vi "Allowed Frequency Mask.vi"() -> ()   [LabVIEW 2010]
panel:
  out "Array":u8[](array[numeric])=[0, 0, 1, 255, 0, 0, 0, 0] format="%.0x"
  out "Allowed Frequencies":u32[](array[numeric])=[70, 75, 80, 85, 90, 95, 100, 110, 120]
  out "Byte #":u8=3
  out "Selected Frequency":u32=70
  in  "ProgramFrequencyIndex":u8=23
  in  "Allowed Frequencies Table {Hz}":cluster{"Bin":u32[], "index":u32[]}[](array[cluster])=[{"Bin"=[14, 12, 10, 8, 6, 4, 3, 2], "index"=[7, 6, 5, 4, 3, 2, 1, 0]}, {"Bin"=[30, 28, 26, 24, 22, 20, 18, 16], "index"=[15, 14, 13, 12, 11, 10, 9, 8]}, {"Bin"=[70, 65, 60, 55, 50, 45, 40, 35], "index"=[23, 22, 21, 20, 19, 18, 17, 16]}, {"Bin"=[120, 110, 100, 95, 90, 85, 80, 75], "index"=[31, 30, 29, 28, 27, 26, 25, 24]}, {"Bin"=[200, 190, 180, 170, 160, 150, 140, 130], "index"=[39, 38, 37, 36, 35, 34, 33, 32]}, {"Bin"=[400, 375, 350, 325, 300, 275, 250, 225], "index"=[47, 46, 45, 44, 43, 42, 41, 40]}, {"Bin"=[1200, 1100, 1000, 900, 800, 700, 600, 500], "index"=[55, 54, 53, 52, 51, 50, 49, 48]}, {"Bin"=[2000, 1900, 1800, 1700, 1600, 1500, 1400, 1300], "index"=[63, 62, 61, 60, 59, 58, 57, 56]}]
  in  "AllowedFrequecies[]":string="0x00, 0x00, 0x01, 0xFF, 0x00, 0x00, 0x00, 0x00"
  # "e.\tAllowedFrequecies[] = 0x00, 0x00, 0xC0, 0xFF, 0x00, 0x00, 0x00, 0x00\nf.\tProgramFrequencyIndex = 23"
  # "0..63 for Patient Stim"
  # "Byte # 1"
  # "Byte # 2"
  # "Byte # 3"
  # "Byte # 4"
  # "Byte # 5"
  # "Byte #6"
  # "Byte # 7"
  # "Byte #8"
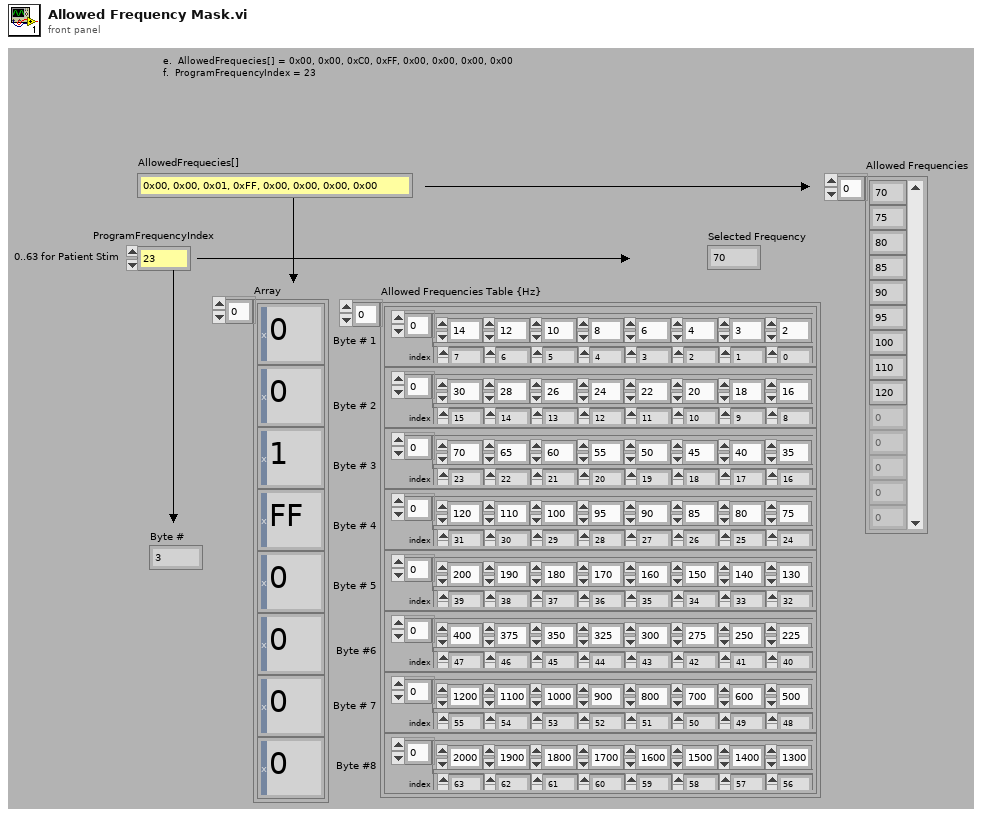
[diagram p1: front panel]
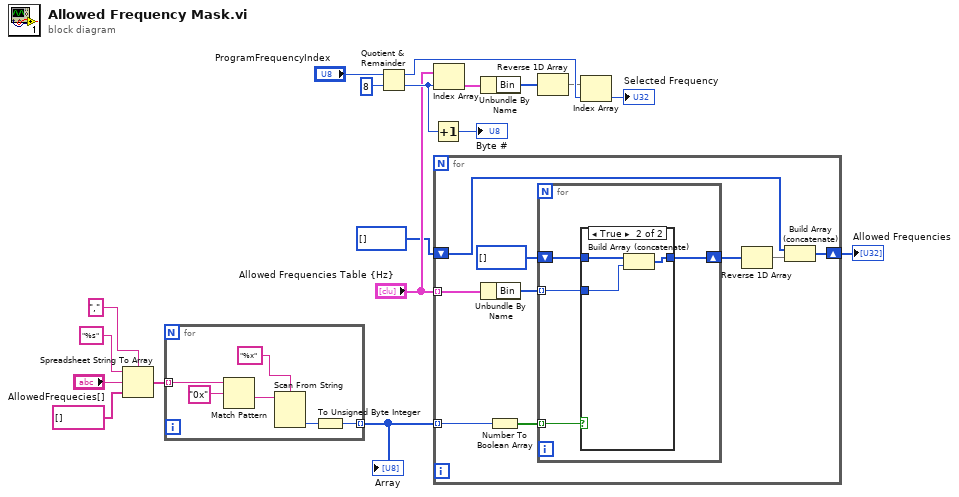
[diagram p0: block diagram]
diagram:
  n1 = Spreadsheet String To Array(delimiter (Tab)=",", format string="%s" ("spreadsheet string"), spreadsheet string="AllowedFrequecies[]", array type (2D Dbl)=string[] []) -> (array=w14:string[])
  n2 = for {
    tunnel: w14 -> [w22] mode=indexing
    tunnel: [w19] -> w4 mode=indexing
    n3 = Match Pattern(string=w22, regular expression="0x" ("format string")) -> (after substring=w20:string)  [unwired: 1 in, 3 out]
    n4 = Scan From String(format string="%x", input string=w20) -> (output 1=w23:i32)  [unwired: 3 in, 3 out]
    n5 = To Unsigned Byte Integer(number=w23) -> (unsigned 8bit integer=w19:u8)
  }
  "Array" <- w4
  n6 = Quotient & Remainder(x="ProgramFrequencyIndex", y=u8 8) -> (x-y*floor(x/y)=w7:u8, floor(x/y)=w10:u8)
  n7 = Increment(x=w10) -> (x+1=→"Byte #":u8)
  n8 = Index Array(array="Allowed Frequencies Table {Hz}", index=w10) -> (element=w9:cluster{"Bin":u32[], "index":u32[]})
  n9 = for {
    tunnel: w4 -> [w33] mode=indexing
    tunnel: "Allowed Frequencies Table {Hz}" -> [w31] mode=indexing
    shift-right: [w25] -> w1
    shift-left: u32[] [] ("Allowed Frequencies") -> [w27]
    n10 = Unbundle By Name(w31) -> ("Bin"=w30:u32[])
    n11 = Number To Boolean Array(number=w33) -> (Boolean array=w32:bool[])
    n12 = for {
      shift-right: [w34] -> w28
      shift-left: u32[] [] ("Allowed Frequencies") -> [w37]
      tunnel: w32 -> [w36] mode=indexing
      tunnel: w30 -> [w35] mode=indexing
      n13 = case shown="True" w36 {
        tunnel: w37 -> [w38 w41]
        tunnel: [w38 w40] -> w34
        tunnel: w35 -> [_ w39]
        frame False {
        }
        frame True {
          n14 = Build Array (concatenate)(w41, w39) -> (w40:u32[])
        }
      }
    }
    n15 = Reverse 1D Array(array=w28) -> (reversed array=w26:u32[])
    n16 = Build Array (concatenate)(w27, w26) -> (w25:u32[])
  }
  "Allowed Frequencies" <- w1
  n17 = Unbundle By Name(w9) -> ("Bin"=w8:u32[])
  n18 = Reverse 1D Array(array=w8) -> (reversed array=w6:u32[])
  n19 = Index Array(array=w6, index=w7) -> (element=→"Selected Frequency":u32)
